vi "CORRH.vi"(9 "Array":i32[](array[numeric])) -> (1 "element":i32)   [LabVIEW 2016]
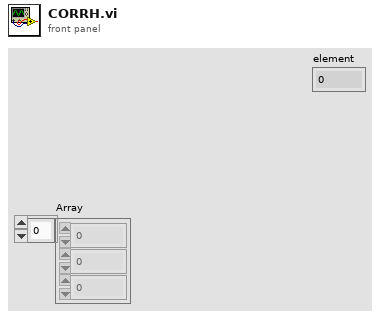
[diagram p1: front panel]
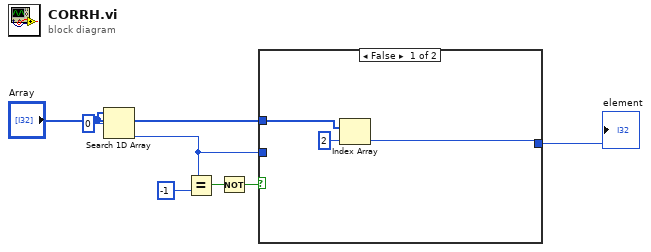
[diagram p0: block diagram]
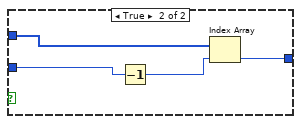
[diagram p2: hidden frame]
diagram:
  n1 = Search 1D Array(1D array="Array", element=0) -> (index of element=w4:i32)  [unwired: 1 in]
  n2 = Equal?(x=w4, y=-1) -> (x = y?=w1:bool)
  n3 = Not(x=w1) -> (.not. x?=w2:bool)
  n4 = case shown="False" w2 {
    tunnel: w4 -> [_ w14]
    tunnel: "Array" -> [w10 w12]
    tunnel: [w8 w11] -> w5
    frame False {
      n5 = Index Array(array=w10, index=2) -> (element=w8:i32)
    }
    frame True {
      n6 = Decrement(x=w14) -> (x-1=w13:i32)
      n7 = Index Array(array=w12, index=w13) -> (element=w11:i32)
    }
  }
  "element" <- w5
